vi "Finish.vi"(4 "error in":errorcluster) -> ()   [LabVIEW 2011]
doc: "This VI is called just before exiting. It is expected to close I/O refnum, save collected data, etc."
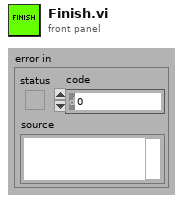
[diagram p1: front panel]
types:
  T1 = typedef "WPI_SolenoidDevRef.ctl" = cluster{"DevStatus":errorcluster, "Solenoid Module":T2, "Forward Solenoid Channel":T3, "Reverse Solenoid Channel":T3}
  T2 = typedef "FPGA_TypedefSolenoidModule.ctl" = enum16{"Solenoid Module 1", "Solenoid Module 2"}
  T3 = typedef "WPI_SolenoidChannel.ctl" = enum8{"Solenoid 1", "Solenoid 2", "Solenoid 3", "Solenoid 4", "Solenoid 5", "Solenoid 6", "Solenoid 7", "Solenoid 8", "Invalid"}
  T4 = typedef "WPI_I2CDevRef.ctl" = cluster{"DevStatus":errorcluster, "Digital Module":T5, "Device Address":u8}
  T5 = typedef "FPGA_TypedefDigitalModule.ctl" = enum16{"Digital Module 1", "Digital Module 2"}
  T6 = typedef "WPI_JoystickDevRef.ctl" = cluster{"Device":T7}
  T7 = typedef "WPI_JoystickDeviceEnum.ctl" = enum16{"USB 1", "USB 2", "USB 3", "USB 4", "Kinect 1", "Kinect 2"}
  T8 = typedef "WPI_CameraDevRef.ctl" = cluster{"Camera Address":string, "CameraStatus":errorcluster, "Acquire Image Notifier":refnum<notifier>}
  T9 = typedef "WPI_RobotDriveDevRef.ctl" = cluster{"DevStatus":errorcluster, "Motors[]":T10[], "Square Inputs":bool, "Max Output":dbl, "Isochronous":bool}
  T10 = typedef "WPI_MotorControlDeviceRef.ctl" = cluster{"DeviceStatus":errorcluster, "Type":enum16{"PWM", "CAN"}, "PWM":cluster{"Digital Module":T5, "PWM Channel":T11, "DeadBand":T12}, "CAN":cluster{"Device Number":u8, "Control Mode":T13, "Semaphore":T14, "Max Vout":dbl}, "Invert":bool, "TransformRef":T15, "InvTransformRef":T15}
  T11 = typedef "FPGA_DIOPWMChannel.ctl" = enum8{"PWM 1", "PWM 2", "PWM 3", "PWM 4", "PWM 5", "PWM 6", "PWM 7", "PWM 8", "PWM 9", "PWM 10", "Invalid"}
  T12 = typedef "WPI_PWMDeadband.ctl" = cluster{"Name":string, "maxPositivePwm":i32, "minPositivePwm":i32, "centerPwm":i32, "maxNegativePwm":i32, "minNegativePwm":i32, "angularRange":u16}
  T13 = typedef "WPI_CANJaguar_ControlMode.ctl" = enum8{"Percent VBus", "Current", "Speed", "Position", "Voltage"}
  T14 = typedef "Semaphore RefNum" = refnum<k1>
  T15 = typedef "WPI_PWMTransform_ConPane.ctl" = refnum<vi>
  T16 = typedef "WPI_EncoderDevRef.ctl" = cluster{"DevStatus":errorcluster, "EncoderIndex":T17, "CounterIndex":T18, "DistancePerCount":dbl, "Decoding Type":T19}
  T17 = typedef "FPGA_EncoderIdx.ctl" = enum8{"Enc 0", "Enc 1", "Enc 2", "Enc 3", "Invalid"}
  T18 = typedef "FPGA_CounterCtrSystemIndex.ctl" = enum8{"Ctr 0", "Ctr 1", "Ctr 2", "Ctr 3", "Ctr 4", "Ctr 5", "Ctr 6", "Ctr 7", "Invalid"}
  T19 = typedef "WPI_EncoderType.ctl" = enum16{"1x", "2x", "4x"}
  T20 = typedef "WPI_GyroDevRef.ctl" = cluster{"DevStatus":errorcluster, "Analog Module":T21, "Analog Channel":T22, "Offset":dbl, "Gain (VoltsPerDegree/Second)":dbl}
  T21 = typedef "FPGA_TypedefAnalogModule.ctl" = enum16{"Analog Module 1", "Analog Module 2"}
  T22 = typedef "FPGA_AIChannel.ctl" = enum8{"AI 1", "AI 2", "AI 3", "AI 4", "AI 5", "AI 6", "AI 7", "AI 8", "Invalid"}
  T23 = typedef "WPI_DigitalInputDevRef.ctl" = cluster{"DevStatus":errorcluster, "DIO Channel":T24, "Digital Module":T5}
  T24 = typedef "FPGA_DIOChannel.ctl" = enum8{"DIO 1", "DIO 2", "DIO 3", "DIO 4", "DIO 5", "DIO 6", "DIO 7", "DIO 8", "DIO 9", "DIO 10", "DIO 11", "DIO 12", "DIO 13", "DIO 14", "Invalid"}
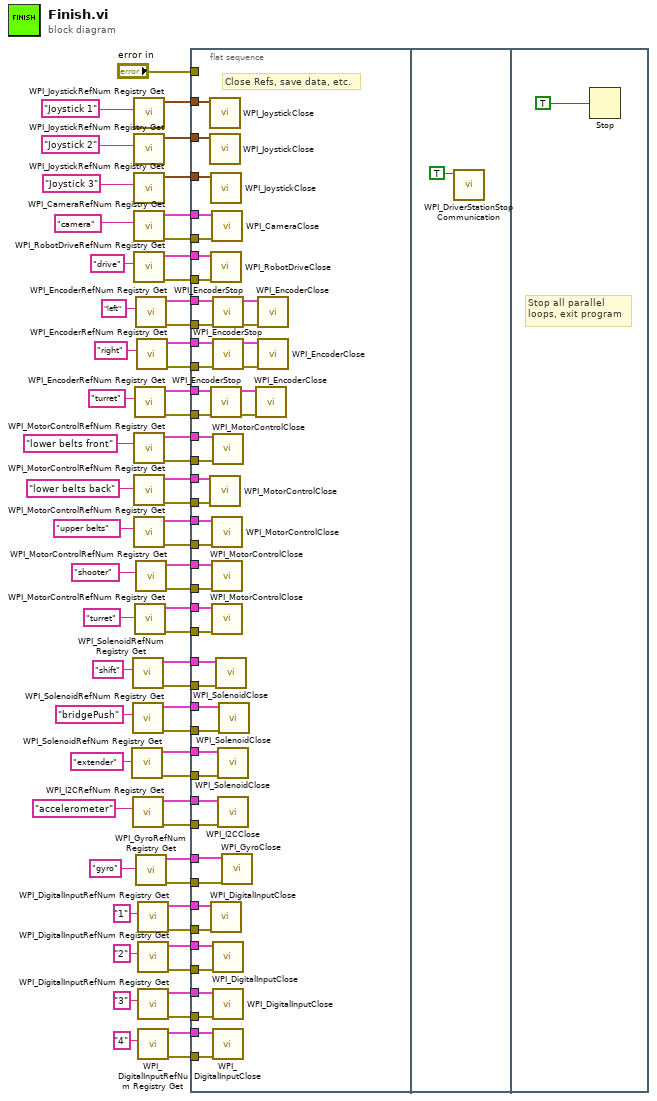
[diagram p0: block diagram]
diagram:
  n1 = call <vilib>:"WPI_SolenoidRefNum Registry Get.vi"("refnum name"="extender") -> ("error out"=w13:errorcluster, "SolenoidDevRef"=w14:T1)  [unwired: 9 in]
  n2 = call <vilib>:"WPI_SolenoidRefNum Registry Get.vi"("refnum name"="shift") -> ("error out"=w27:errorcluster, "SolenoidDevRef"=w28:T1)  [unwired: 9 in]
  n3 = call <vilib>:"WPI_SolenoidRefNum Registry Get.vi"("refnum name"="bridgePush") -> ("error out"=w23:errorcluster, "SolenoidDevRef"=w24:T1)  [unwired: 9 in]
  n4 = call <vilib>:"WPI_I2CRefNum Registry Get.vi"("refnum name"="accelerometer") -> ("error out"=w20:errorcluster, "I2CDevRef"=w21:T4)  [unwired: 9 in]
  n5 = call <vilib>:"WPI_JoystickRefNum Registry Get.vi"("refnum name"="Joystick 1") -> ("JoystickDevRef"=w63:T6)  [unwired: 1 in, 9 out]
  n6 = call <vilib>:"WPI_JoystickRefNum Registry Get.vi"("refnum name"="Joystick 2") -> ("JoystickDevRef"=w60:T6)  [unwired: 1 in, 9 out]
  n7 = call <vilib>:"WPI_JoystickRefNum Registry Get.vi"("refnum name"="Joystick 3") -> ("JoystickDevRef"=w57:T6)  [unwired: 1 in, 9 out]
  n8 = call <vilib>:"WPI_CameraRefNum Registry Get.vi"("refnum name"="camera") -> ("error out"=w50:errorcluster, "CameraDevRef"=w62:T8)  [unwired: 1 in, 8 out]
  n9 = call <vilib>:"WPI_RobotDriveRefNum Registry Get.vi"("refnum name"="drive") -> ("error out"=w49:errorcluster, "RobotDriveDevRef"=w55:T9)  [unwired: 9 in]
  n10 = call <vilib>:"WPI_MotorControlRefNum Registry Get.vi"("refnum name"="lower belts front") -> ("error out"=w37:errorcluster, "MotorControlDevRef"=w38:T10)  [unwired: 9 in]
  n11 = call <vilib>:"WPI_MotorControlRefNum Registry Get.vi"("refnum name"="lower belts back") -> ("error out"=w35:errorcluster, "MotorControlDevRef"=w36:T10)  [unwired: 9 in]
  n12 = call <vilib>:"WPI_MotorControlRefNum Registry Get.vi"("refnum name"="upper belts") -> ("error out"=w33:errorcluster, "MotorControlDevRef"=w34:T10)  [unwired: 9 in]
  n13 = call <vilib>:"WPI_EncoderRefNum Registry Get.vi"("refnum name"="turret") -> ("error out"=w46:errorcluster, "EncoderDevRef"=w44:T16)  [unwired: 9 in]
  n14 = call <vilib>:"WPI_MotorControlRefNum Registry Get.vi"("refnum name"="turret") -> ("error out"=w29:errorcluster, "MotorControlDevRef"=w30:T10)  [unwired: 9 in]
  n15 = call <vilib>:"WPI_EncoderRefNum Registry Get.vi"("refnum name"="left") -> ("error out"=w48:errorcluster, "EncoderDevRef"=w52:T16)  [unwired: 9 in]
  n16 = call <vilib>:"WPI_MotorControlRefNum Registry Get.vi"("refnum name"="shooter") -> ("error out"=w31:errorcluster, "MotorControlDevRef"=w32:T10)  [unwired: 9 in]
  n17 = call <vilib>:"WPI_GyroRefNum Registry Get.vi"("refnum name"="gyro") -> ("error out"=w17:errorcluster, "GyroDevRef"=w18:T20)  [unwired: 9 in]
  n18 = call <vilib>:"WPI_EncoderRefNum Registry Get.vi"("refnum name"="right") -> ("error out"=w47:errorcluster, "EncoderDevRef"=w51:T16)  [unwired: 9 in]
  n19 = call <vilib>:"WPI_DigitalInputRefNum Registry Get.vi"("refnum name"="1") -> ("error out"=w7:errorcluster, "DigitalInputDevRef"=w8:T23)  [unwired: 9 in]
  n20 = call <vilib>:"WPI_DigitalInputRefNum Registry Get.vi"("refnum name"="2") -> ("error out"=w5:errorcluster, "DigitalInputDevRef"=w6:T23)  [unwired: 9 in]
  n21 = call <vilib>:"WPI_DigitalInputRefNum Registry Get.vi"("refnum name"="3") -> ("error out"=w3:errorcluster, "DigitalInputDevRef"=w4:T23)  [unwired: 9 in]
  n22 = call <vilib>:"WPI_DigitalInputRefNum Registry Get.vi"("refnum name"="4") -> ("error out"=w1:errorcluster, "DigitalInputDevRef"=w2:T23)  [unwired: 9 in]
  n23 = flat-sequence {
    tunnel: w63 -> [w111]
    tunnel: w62 -> [w110]
    tunnel: w60 -> [w109]
    tunnel: w57 -> [w108]
    tunnel: w55 -> [w107]
    tunnel: w52 -> [w106]
    tunnel: w51 -> [w99]
    tunnel: w50 -> [w103]
    tunnel: w49 -> [w102]
    tunnel: w48 -> [w101]
    tunnel: w47 -> [w100]
    tunnel: w46 -> [w95]
    tunnel: w44 -> [w94]
    tunnel: w38 -> [w92]
    tunnel: w37 -> [w91]
    tunnel: w36 -> [w83]
    tunnel: w35 -> [w90]
    tunnel: w34 -> [w84]
    tunnel: w33 -> [w89]
    tunnel: w32 -> [w85]
    tunnel: w31 -> [w88]
    tunnel: w30 -> [w86]
    tunnel: w29 -> [w87]
    tunnel: w28 -> [w81]
    tunnel: w27 -> [w82]
    tunnel: w24 -> [w79]
    tunnel: w23 -> [w80]
    tunnel: w21 -> [w77]
    tunnel: w20 -> [w78]
    tunnel: w18 -> [w75]
    tunnel: w17 -> [w76]
    tunnel: "error in" -> [_]
    tunnel: w14 -> [w73]
    tunnel: w13 -> [w74]
    tunnel: w8 -> [w68]
    tunnel: w7 -> [w69]
    tunnel: w6 -> [w67]
    tunnel: w5 -> [w70]
    tunnel: w4 -> [w66]
    tunnel: w3 -> [w71]
    tunnel: w2 -> [w65]
    tunnel: w1 -> [w72]
    frame #0 {
      # "Close Refs, save data, etc."
      n24 = call <vilib>:"WPI_JoystickClose.vi"("JoystickDevRef"=w111) -> ()  [unwired: 11 out]
      n25 = call <vilib>:"WPI_JoystickClose.vi"("JoystickDevRef"=w109) -> ()  [unwired: 11 out]
      n26 = call <vilib>:"WPI_MotorControlClose.vi"("error in (no error)"=w90, "MotorControlDevRef"=w83) -> ()  [unwired: 9 in, 1 out]
      n27 = call <vilib>:"WPI_JoystickClose.vi"("JoystickDevRef"=w108) -> ()  [unwired: 11 out]
      n28 = call <vilib>:"WPI_RobotDriveClose.vi"("error in (no error)"=w102, "RobotDriveDevRef"=w107) -> ()  [unwired: 9 in, 1 out]
      n29 = call <vilib>:"WPI_EncoderStop.vi"("error in (no error)"=w95, "EncoderDevRef"=w94) -> ("error out"=w96:errorcluster, "EncoderDevRef"=w93:T16)  [unwired: 8 in]
      n30 = call <vilib>:"WPI_DigitalInputClose.vi"("error in (no error)"=w69, "DigitalInputDevRef"=w68) -> ()  [unwired: 9 in, 1 out]
      n31 = call <vilib>:"WPI_CameraClose.vi"("error in (no error)"=w103, "CameraDevRef"=w110) -> ()  [unwired: 10 out]
      n32 = call <vilib>:"WPI_MotorControlClose.vi"("error in (no error)"=w89, "MotorControlDevRef"=w84) -> ()  [unwired: 9 in, 1 out]
      n33 = call <vilib>:"WPI_MotorControlClose.vi"("error in (no error)"=w88, "MotorControlDevRef"=w85) -> ()  [unwired: 9 in, 1 out]
      n34 = call <vilib>:"WPI_MotorControlClose.vi"("error in (no error)"=w87, "MotorControlDevRef"=w86) -> ()  [unwired: 9 in, 1 out]
      n35 = call <vilib>:"WPI_EncoderStop.vi"("error in (no error)"=w101, "EncoderDevRef"=w106) -> ("error out"=w105:errorcluster, "EncoderDevRef"=w104:T16)  [unwired: 8 in]
      n36 = call <vilib>:"WPI_EncoderStop.vi"("error in (no error)"=w100, "EncoderDevRef"=w99) -> ("error out"=w97:errorcluster, "EncoderDevRef"=w98:T16)  [unwired: 8 in]
      n37 = call <vilib>:"WPI_MotorControlClose.vi"("error in (no error)"=w91, "MotorControlDevRef"=w92) -> ()  [unwired: 9 in, 1 out]
      n38 = call <vilib>:"WPI_DigitalInputClose.vi"("error in (no error)"=w70, "DigitalInputDevRef"=w67) -> ()  [unwired: 9 in, 1 out]
      n39 = call <vilib>:"WPI_DigitalInputClose.vi"("error in (no error)"=w71, "DigitalInputDevRef"=w66) -> ()  [unwired: 9 in, 1 out]
      n40 = call <vilib>:"WPI_DigitalInputClose.vi"("error in (no error)"=w72, "DigitalInputDevRef"=w65) -> ()  [unwired: 9 in, 1 out]
      n41 = call <vilib>:"WPI_SolenoidClose.vi"("error in (no error)"=w82, "SolenoidDevRef"=w81) -> ()  [unwired: 9 in, 1 out]
      n42 = call <vilib>:"WPI_SolenoidClose.vi"("error in (no error)"=w74, "SolenoidDevRef"=w73) -> ()  [unwired: 9 in, 1 out]
      n43 = call <vilib>:"WPI_I2CClose.vi"("error in (no error)"=w78, "I2CDevRef"=w77) -> ()  [unwired: 9 in, 1 out]
      n44 = call <vilib>:"WPI_SolenoidClose.vi"("error in (no error)"=w80, "SolenoidDevRef"=w79) -> ()  [unwired: 9 in, 1 out]
      n45 = call <vilib>:"WPI_GyroClose.vi"("error in (no error)"=w76, "GyroDevRef"=w75) -> ()  [unwired: 9 in, 1 out]
      n46 = call <vilib>:"WPI_EncoderClose.vi"("error in (no error)"=w96, "EncoderDevRef"=w93) -> ()  [unwired: 9 in, 1 out]
      n47 = call <vilib>:"WPI_EncoderClose.vi"("error in (no error)"=w105, "EncoderDevRef"=w104) -> ()  [unwired: 9 in, 1 out]
      n48 = call <vilib>:"WPI_EncoderClose.vi"("error in (no error)"=w97, "EncoderDevRef"=w98) -> ()  [unwired: 9 in, 1 out]
    }
    frame #1 {
      n49 = call <vilib>:"WPI_DriverStationStop Communication.vi"("StopCommunication"=TRUE) -> ()  [unwired: 10 in, 1 out]
    }
    frame #2 {
      # "Stop all parallel\nloops, exit program"
      n50 = Stop(stop? (T)=TRUE ("Quit")) -> ()
    }
  }
